vi "extract_avg_data.vi"(2 "Combo Box":string(combo), 7 "avg_Q_data in":T2) -> (8 "avg_Q_data out":T2, 12 "RT Avg Data Out":T3, 14 "Summed Avg Data":T1, 15 "error out":errorcluster)   [LabVIEW 2023]
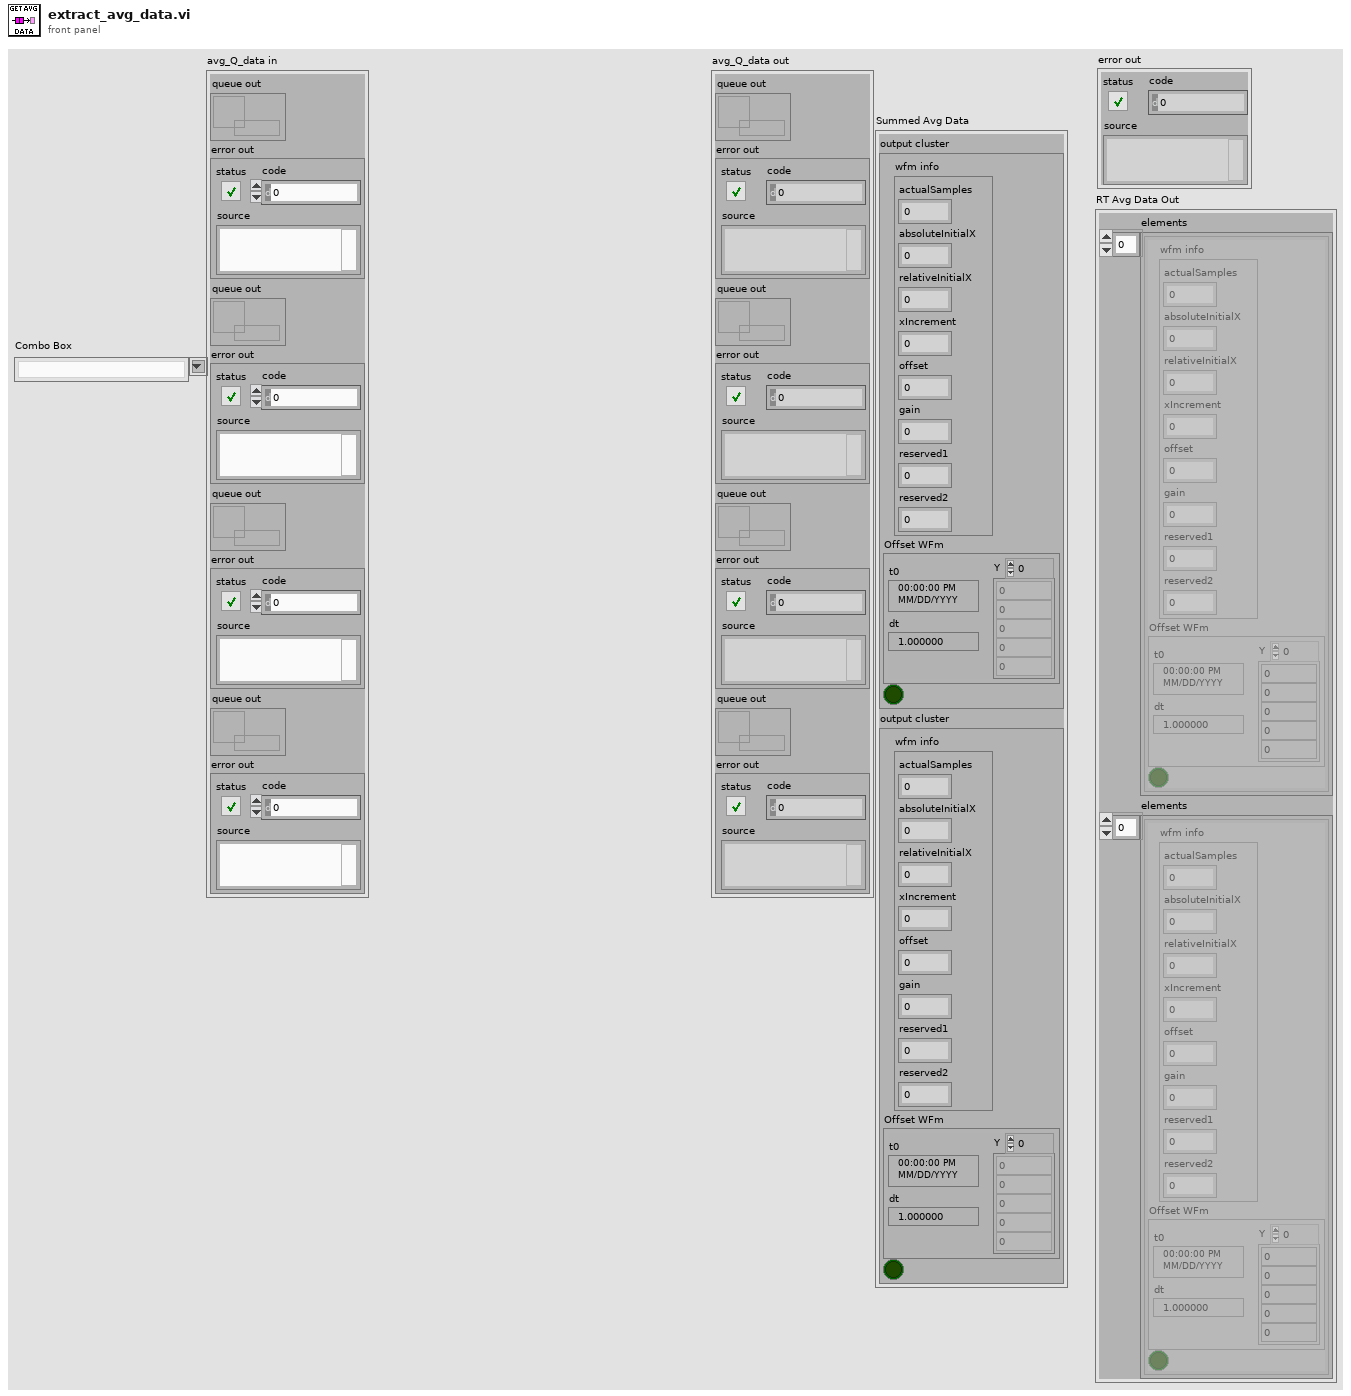
[diagram p1: front panel]
types:
  T1 = cluster{"output cluster":cluster{"wfm info":cluster{"actualSamples":i32, "absoluteInitialX":dbl, "relativeInitialX":dbl, "xIncrement":dbl, "offset":dbl, "gain":dbl, "reserved1":dbl, "reserved2":dbl}, "Offset WFm":waveform(dbl), bool}, "output cluster":cluster{"wfm info":cluster{"actualSamples":i32, "absoluteInitialX":dbl, "relativeInitialX":dbl, "xIncrement":dbl, "offset":dbl, "gain":dbl, "reserved1":dbl, "reserved2":dbl}, "Offset WFm":waveform(dbl), bool}}
  T2 = cluster{"queue out":refnum<queue>, "error out":errorcluster, "queue out":refnum<queue>, "error out":errorcluster, "queue out":refnum<queue>, "error out":errorcluster, "queue out":refnum<queue>, "error out":errorcluster}
  T3 = cluster{"elements":cluster{"wfm info":cluster{"actualSamples":i32, "absoluteInitialX":dbl, "relativeInitialX":dbl, "xIncrement":dbl, "offset":dbl, "gain":dbl, "reserved1":dbl, "reserved2":dbl}, "Offset WFm":waveform(dbl), bool}[], "elements":cluster{"wfm info":cluster{"actualSamples":i32, "absoluteInitialX":dbl, "relativeInitialX":dbl, "xIncrement":dbl, "offset":dbl, "gain":dbl, "reserved1":dbl, "reserved2":dbl}, "Offset WFm":waveform(dbl), bool}[]}
  T4 = cluster{"wfm info":cluster{"actualSamples":i32, "absoluteInitialX":dbl, "relativeInitialX":dbl, "xIncrement":dbl, "offset":dbl, "gain":dbl, "reserved1":dbl, "reserved2":dbl}, "Offset WFm":waveform(dbl), bool}[]
  T5 = cluster{"wfm info":cluster{"actualSamples":i32, "absoluteInitialX":dbl, "relativeInitialX":dbl, "xIncrement":dbl, "offset":dbl, "gain":dbl, "reserved1":dbl, "reserved2":dbl}, "Offset WFm":waveform(dbl), bool}
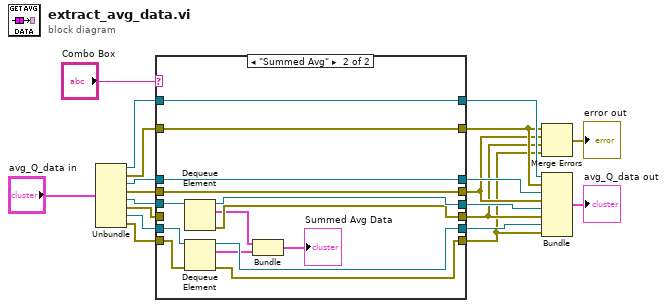
[diagram p0: block diagram]
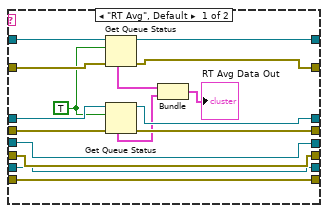
[diagram p2: hidden frame]
diagram:
  n1 = Unbundle("avg_Q_data in") -> ("queue out"=w20:refnum<queue>, "error out"=w19:errorcluster, "queue out"=w18:refnum<queue>, "error out"=w17:errorcluster, "queue out"=w16:refnum<queue>, "error out"=w15:errorcluster, "queue out"=w14:refnum<queue>, "error out"=w13:errorcluster)
  n2 = case shown="\"Summed Avg\"" "Combo Box" {
    tunnel: w20 -> [w36 w50]
    tunnel: w19 -> [w35 w49]
    tunnel: w18 -> [w34 w48]
    tunnel: w17 -> [w33 w47]
    tunnel: w16 -> [w29 w46]
    tunnel: w15 -> [w28 _]
    tunnel: w14 -> [w26 w45]
    tunnel: w13 -> [w25 w44]
    tunnel: [w32 w50] -> w12
    tunnel: [w31 w49] -> w7
    tunnel: [w30 w48] -> w11
    tunnel: [w29 w41] -> w10
    tunnel: [w28 w40] -> w5
    tunnel: [w27 w47] -> w6
    tunnel: [w26 w43] -> w9
    tunnel: [w25 w42] -> w4
    frame "RT Avg", Default {
      w22 = TRUE ("return elements? (F)")
      n3 = Get Queue Status(queue=w36, return elements? (F)=w22, error in (no error)=w35) -> (queue out=w32:refnum<queue>, error out=w31:errorcluster, elements=w24:T4)  [unwired: 5 out]
      n4 = Get Queue Status(queue=w34, return elements? (F)=w22, error in (no error)=w33) -> (queue out=w30:refnum<queue>, error out=w27:errorcluster, elements=w23:T4)  [unwired: 5 out]
      n5 = Bundle("elements"=w24, "elements"=w23) -> (→"RT Avg Data Out":T3)  [unwired: 1 in]
    }
    frame "Summed Avg" {
      n6 = Dequeue Element(queue=w46) -> (queue out=w41:refnum<queue>, element=w39:T5, error out=w40:errorcluster)  [unwired: 2 in, 1 out]
      n7 = Dequeue Element(queue=w45, error in (no error)=w44) -> (queue out=w43:refnum<queue>, element=w38:T5, error out=w42:errorcluster)  [unwired: 1 in, 1 out]
      n8 = Bundle("output cluster"=w39, "output cluster"=w38) -> (→"Summed Avg Data":T1)  [unwired: 1 in]
    }
  }
  n9 = Merge Errors(w7, w6, w5, w4) -> (→"error out":errorcluster)
  n10 = Bundle("queue out"=w12, "error out"=w7, "queue out"=w11, "error out"=w6, "queue out"=w10, "error out"=w5, "queue out"=w9, "error out"=w4) -> (→"avg_Q_data out":T2)  [unwired: 1 in]
